vi "FTW-Actor-Log-Event.vi"(0 "FTW Actor Instance":refnum<class "FTW-Actor-Instance.lvclass">, 5 "Event Type":string, 7 "Event Data":string, 11 "error in":errorcluster) -> (4 "FTW Actor Instance out":refnum<class "FTW-Actor-Instance.lvclass">, 6 "Serialized Event":string, 15 "error out":errorcluster)   [LabVIEW 2013, in "FTW-Actor-Instance.lvclass"]
uses:
  FTW-Actor-Instance.lvclass
  FTW-Actor-Instance.lvclass/FTW-Actor-Instance.ctl
  logger/FTW-Logger.lvclass
panel:
  # "Inputs"
  # "Outputs"
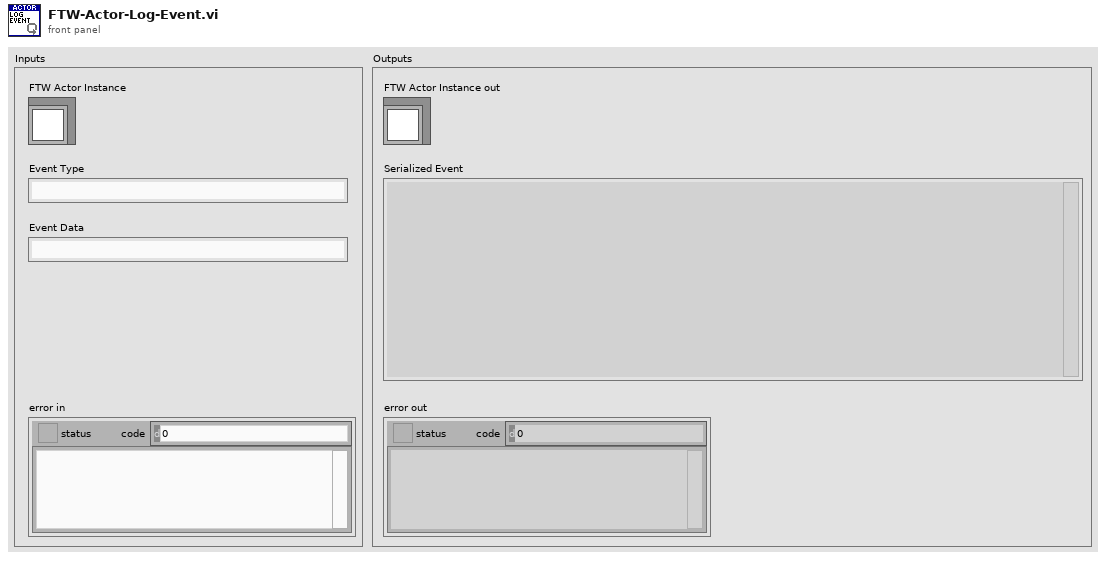
[diagram p1: front panel]
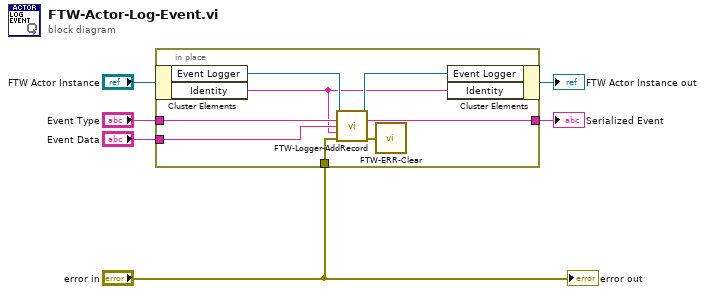
[diagram p0: block diagram]
diagram:
  n1 = in-place {
    in-place-border: "error in" -> [w14]
    in-place-border: [w11] -> w4
    in-place-border: "Event Type" -> [w10]
    in-place-border: "Event Data" -> [w9]
    n2 = in-place-cluster #1("FTW Actor Instance") -> ("Event Logger"=w13:refnum<class "FTW-Logger.lvclass">, "Identity"=w8:string)
    n3 = call "FTW-Logger-AddRecord.vi"("FTW Logger Connector"=w13, "Event Type"=w10, "Event Data"=w9, "Source (unwired for call chain)"=w8, "error in"=w14) -> ("FTW Logger Connector out"=w12:refnum<class "FTW-Logger.lvclass">, "Serialized Event"=w11:string, "error out"=w7:errorcluster)  [unwired: 8 in]
    n4 = call "FTW-ERR-Clear.vi"("error to snuff"=w7) -> ()  [unwired: 1 out]
    n5 = in-place-cluster #1("Event Logger"=w12, "Identity"=w8) -> (→"FTW Actor Instance out":refnum<class "FTW-Actor-Instance.lvclass">)
  }
  "Serialized Event" <- w4
  "error out" <- "error in"
